vi "Open.vi"(8 "error in (no error)":errorcluster, 10 "address":string, 11 "RP100 in":refnum<class "RP100.lvclass">) -> (0 "error out":errorcluster, 3 "RP100 out":refnum<class "RP100.lvclass">)   [LabVIEW 2019, in "RP100.lvclass"]
uses:
  RP100.lvclass
  C:/Program Files (x86)/National Instruments/LabVIEW 2019/user.lib/LevyLab/Levylab Instruments/SMOs/Instrument/Instrument.lvclass
  <userlib>/LevyLab/Instrument Framework/Instrument Types/Strain/Instrument.Strain.lvclass
  <userlib>/LevyLab/Instrument Framework/SMOs/Instrument/Instrument.lvclass
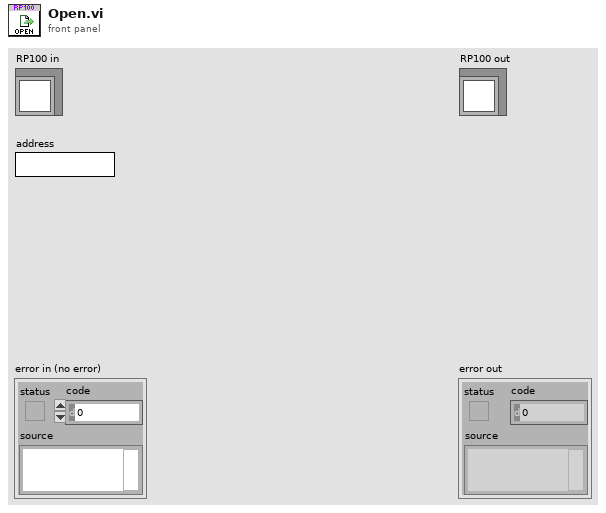
[diagram p1: front panel]
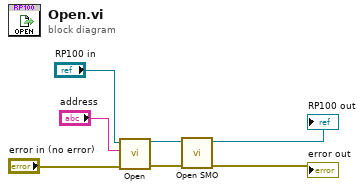
[diagram p0: block diagram]
diagram:
  n1 = call-parent "Open.vi"("error in (no error)"="error in (no error)", "address"="address", "Instrument in"="RP100 in") -> ("error out"=w3:errorcluster, "Instrument out"=w4:refnum<class "RP100.lvclass">)  [unwired: 7 in]
  n2 = call <userlib>:"Open SMO.vi"("error in (no error)"=w3, "Instrument in"=w4) -> ("error out"=→"error out":errorcluster, "Instrument out"=→"RP100 out":refnum<class "RP100.lvclass">)  [unwired: 8 in]
